vi "Initialize.vi"(8 "error in":errorcluster, 9 "LimitExpression":string, 10 "Name":string, 11 "MeasureLimit in":refnum<class "MeasureLimit.lvclass">) -> (0 "error out":errorcluster, 3 "MeasureLimit out":refnum<class "MeasureLimit.lvclass">)   [LabVIEW 2021, in "ProligentXMLGenerator.lvlib" / "MeasureLimit.lvclass"]
uses:
  MeasureLimit.lvclass
  MeasureLimit.lvclass/MeasureLimit.ctl
  Model/CustomData/CustomData.lvclass
  Base/NonEmptyString_2000/NonEmptyString_2000.lvclass
  Data.ctl
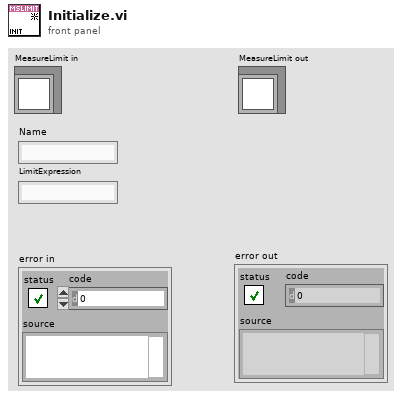
[diagram p1: front panel]
types:
  T1 = typedef "ProligentXMLGenerator.lvlib/MeasureLimit.lvclass/Data.ctl" = cluster{"Name":string, "CustomData":refnum<class "CustomData.lvclass">, "LimitExpression":refnum<class "NonEmptyString_2000.lvclass">}
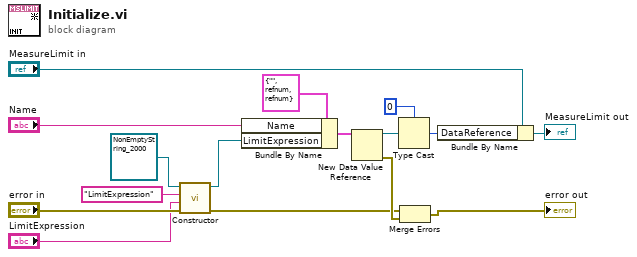
[diagram p0: block diagram]
diagram:
  n1 = call-dynamic "Constructor.vi"("error in"="error in", "Value"="LimitExpression", "Name"="LimitExpression", "String in"=refnum<class "NonEmptyString_2000.lvclass"> refnum ("ProligentCanonicalFile:Guid.lvclass")) -> ("error out"=w5:errorcluster, "String out"=w2:refnum<class "NonEmptyString_2000.lvclass">)  [unwired: 6 in]
  n2 = Bundle By Name(cluster=T1 {"Name"="", "CustomData"=refnum, "LimitExpression"=refnum} ("Data"), "Name"="Name", "LimitExpression"=w2) -> (w12:T1)
  n3 = New Data Value Reference(data value=w12) -> (data value reference=w13:refnum<data-value>, error out=w16:errorcluster)  [unwired: 1 in]
  n4 = Type Cast(type=u64 0, x=w13) -> (*(type *) &x=w15:u64)
  n5 = Merge Errors(w5, w16) -> (→"error out":errorcluster)
  n6 = Bundle By Name(cluster="MeasureLimit in", "DataReference"=w15) -> (→"MeasureLimit out":refnum<class "MeasureLimit.lvclass">)
